vi "form_3D_data.vi"(9 "z data":dbl[](array[numeric]), 10 "y data":dbl[](array[numeric]), 11 "x data":dbl[](array[numeric])) -> (1 "Z matrix":dbl[][](array[numeric]), 2 "y vector":dbl[](array[numeric]), 3 "x vector":dbl[](array[numeric]))   [LabVIEW 2018]
doc: "MeasGUI - Measurement Graphics User Interface\nCopyright (c) 2018 Frans Korhonen\n\nMeasGUI was originally developed at Institute for Atmospheric \nand Earth System Research / Physics, Faculty of Science, \nUniversity of Helsinki, Finland\n\nAssistance, experience and feedback from following persons have been \ncritical in development of MeasGUI: Michel Attoui, Juha Kangasluoma, \nLauri Ahonen, Ella Häkkinen, Markku Kulmala and Tuukka Petäjä.\n\nThis file is part of MeasGUI.\n\nThis Source Code Form is subject to the terms of the Mozilla Public\nLicense, v. 2.0. If a copy of the MPL was not distributed with this\nfile, You can obtain one at http://mozilla.org/MPL/2.0/."
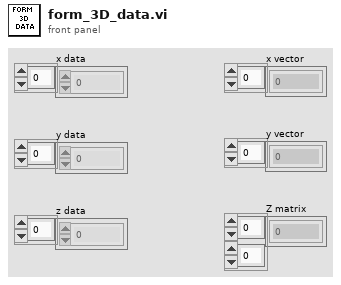
[diagram p1: front panel]
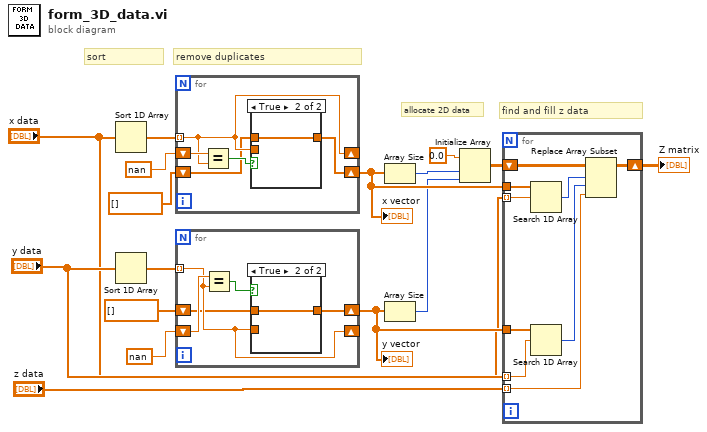
[diagram p0: block diagram]
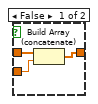
[diagram p2: hidden frame]
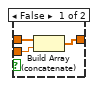
[diagram p3: hidden frame]
diagram:
  # "allocate 2D data"
  # "find and fill z data"
  # "sort"
  # "remove duplicates"
  n1 = Sort 1D Array(array="x data") -> (sorted array=w16:dbl[])
  n2 = Sort 1D Array(array="y data") -> (sorted array=w3:dbl[])
  n3 = for {
    tunnel: w16 -> [w19] mode=indexing
    shift-right: [w19] -> _
    shift-left: nan ("Numeric") -> [w21]
    shift-right: [w18] -> w13
    shift-left: dbl[] [] -> [w17]
    n4 = Equal?(x=w21, y=w19) -> (x = y?=w20:bool)
    n5 = case shown="True" w20 {
      tunnel: w19 -> [w23 _]
      tunnel: [w24 w25] -> w18
      tunnel: w17 -> [w22 w25]
      frame False {
        n6 = Build Array (concatenate)(w22, w23) -> (w24:dbl[])
      }
      frame True {
      }
    }
  }
  "x vector" <- w13
  n7 = for {
    tunnel: w3 -> [w28] mode=indexing
    shift-right: [w28] -> _
    shift-left: nan ("Numeric") -> [w30]
    shift-right: [w27] -> w14
    shift-left: dbl[] [] -> [w26]
    n8 = Equal?(x=w30, y=w28) -> (x = y?=w29:bool)
    n9 = case shown="True" w29 {
      tunnel: w28 -> [w32 _]
      tunnel: [w33 w34] -> w27
      tunnel: w26 -> [w31 w34]
      frame False {
        n10 = Build Array (concatenate)(w31, w32) -> (w33:dbl[])
      }
      frame True {
      }
    }
  }
  "y vector" <- w14
  n11 = Array Size(array=w13) -> (size(s)=w8:i32)
  n12 = Array Size(array=w14) -> (size(s)=w7:i32)
  n13 = Initialize Array(0.0 ("element"), w8, w7) -> (w12:dbl[][])
  n14 = for {
    tunnel: "x data" -> [w43] mode=indexing
    tunnel: w14 -> [w41]
    tunnel: w13 -> [w42]
    tunnel: "y data" -> [w40] mode=indexing
    tunnel: "z data" -> [w35] mode=indexing
    shift-right: [w36] -> w15
    shift-left: w12 -> [w37]
    n15 = Search 1D Array(1D array=w42, element=w43) -> (index of element=w39:i32)  [unwired: 1 in]
    n16 = Search 1D Array(1D array=w41, element=w40) -> (index of element=w38:i32)  [unwired: 1 in]
    n17 = Replace Array Subset(array=w37, new element=w35, index (row)=w39, index (col)=w38) -> (w36:dbl[][])
  }
  "Z matrix" <- w15
